vi "Test Settings.vi"() -> ()   [LabVIEW 2016, in "Hall Effect Library.lvlib"]
uses:
  Hall Effect Library.lvlib
  Public/Controls/Resisitivity.ctl
panel:
  out "Slot Number of 3765 Card":u32
  in  "Sample Width Ws":dbl
  in  "Sample Dimensions D2":dbl
  in  "Sample Dimensions D1":dbl
  in  "Sample dimensions y":dbl
  in  "Sample dimensions x":dbl
  in  "Count Voltmeter":i32=1 min=1 max=1024
  in  "NPLC Voltmeter":dbl=1.0 min=0.001 max=10.0
  in  "Count Ammeter":i32=1 min=1 max=1024
  in  "NPLC Ammeter":dbl=1.0 min=0.001 max=10.0
  in  "Magnetic Flux":dbl
  in  "Sample Thickness":dbl
  in  "Soak Time":dbl
  in  "Current Level":dbl
  in  "Voltage Limit":dbl
  in  "Resistivity":T1
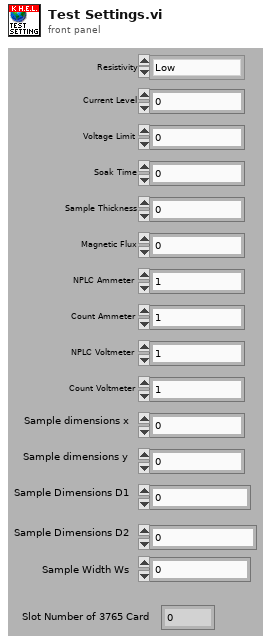
[diagram p1: front panel]
types:
  T1 = typedef "Hall Effect Library.lvlib/Resisitivity.ctl" = enum16{"Low", "High"}
diagram:
